vi "Get Date String.vi"(8 "error in (no error)":errorcluster, 11 "Type A In":refnum<class "Type B.lvclass">) -> (0 "error out":errorcluster, 2 "Date String":string, 3 "Type A Out":refnum<class "Type B.lvclass">)   [LabVIEW 2020, in "Barcode Reader Second Iteration.lvlib" / "Type B.lvclass"]
uses:
  Type B.lvclass
  Type B.lvclass/Type B.ctl
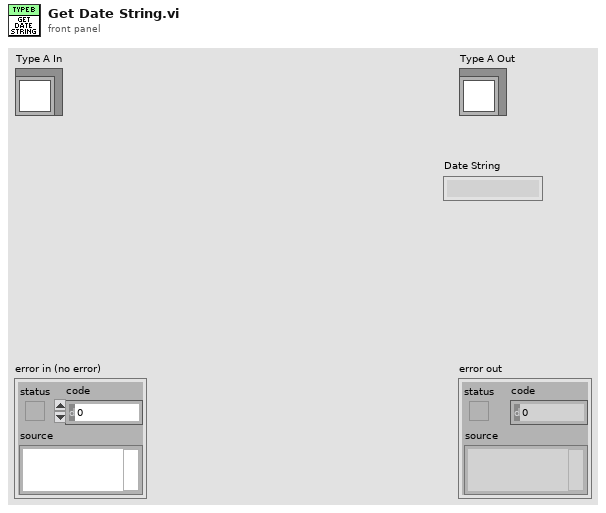
[diagram p1: front panel]
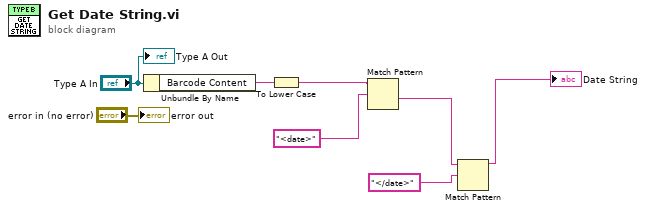
[diagram p0: block diagram]
diagram:
  n1 = Unbundle By Name("Type A In") -> ("Barcode Content"=w6:string)
  n2 = To Lower Case(string=w6) -> (all lower case string=w1:string)
  n3 = Match Pattern(string=w1, regular expression="<date>" ("format string")) -> (after substring=w4:string)  [unwired: 1 in, 3 out]
  n4 = Match Pattern(string=w4, regular expression="</date>" ("format string")) -> (before substring=→"Date String":string)  [unwired: 1 in, 3 out]
  "error out" <- "error in (no error)"
  "Type A Out" <- "Type A In"
